vi "Mic Amps Sync.vi"() -> ()   [LabVIEW 2018, in "Impedance Tube.lvlib"]
uses:
  <vilib>/sound2/lvsound2.llb/Sound Data Format.ctl
  <vilib>/sound2/lvsound2.llb/Sampling Mode.ctl
  <vilib>/sound2/lvsound2.llb/Sound Output Set Volume (Single).vi
  <vilib>/sound2/lvsound2.llb/Sound Output Write (DBL Single).vi
  <vilib>/sound2/lvsound2.llb/Sound Input Read (DBL).vi
  <vilib>/addons/Sound and Vibration/svt_Level/SVT Sound Level (N Ch).vi
  Impedance Tube.lvlib
  <vilib>/measure/NI_MABase.lvlib
  <vilib>/addons/Sound and Vibration/svt_Level/SoundVib_SoundLevel.lvlib
panel:
  out "Scalar 2":dbl
  out "Scalar":dbl
  out "Filtered Signal 3":dynamicdata(graph) caption="Filtered Signal"
  out "Speaker Device":dbl
  out "Filtered Signal 2":dynamicdata(graph) caption="Filtered Signal"
  out "Mic B Device":dbl
  out "mv 2":dbl
  out "db B":dbl
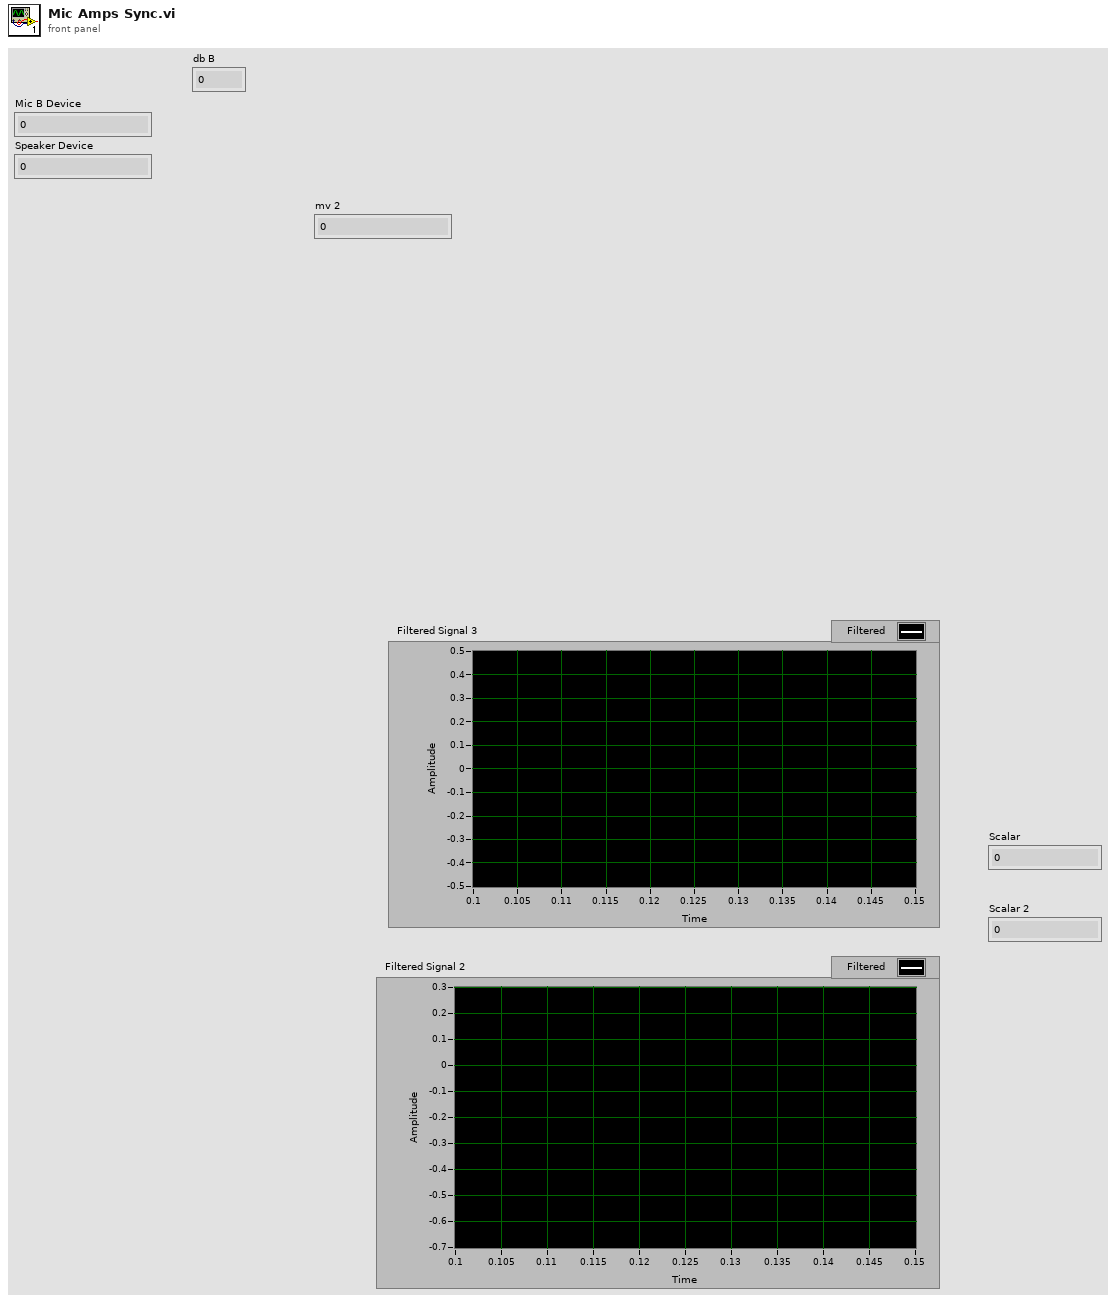
[diagram p1: front panel]
types:
  T1 = cluster{"Leq":bool, "Running Leq":bool, "Exponential":bool, "Peak":bool}
  T2 = typedef "Sound Data Format.ctl" = cluster{"sample rate (S/s)":dbl, "number of channels":i32, "bits per sample":i32}
  T3 = typedef "Sampling Mode.ctl" = i32
  T4 = typedef "Sound Output Task ID.ctl" = u32
  T5 = typedef "Sound Input Task ID.ctl" = u32
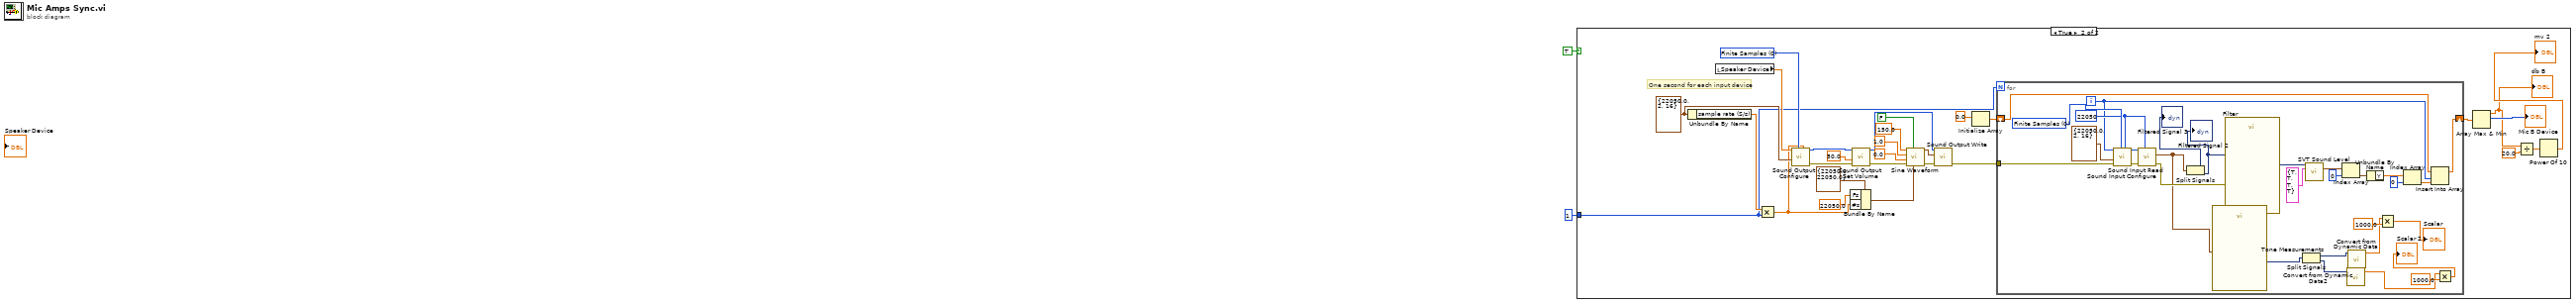
[diagram p0: block diagram]
diagram:
  n1 = case shown="True" TRUE {
    tunnel: 1 ("Number of Input Devices") -> [_ w8]
    frame False {
    }
    frame True {
      w31 = T3 0 items=["Finite Samples", "Continuous Samples"] ("sample mode")
      w18 = T2 {"sample rate (S/s)"=22050.0, "number of channels"=2, "bits per sample"=16} ("sound format")
      # "One second for each input device"
      n2 = Unbundle By Name(w18) -> ("sample rate (S/s)"=w17:dbl)
      n3 = local read "Speaker Device"() -> (w28:dbl)
      n4 = Multiply(x=w17, y=w8) -> (x*y=w15:dbl)
      n5 = call <vilib>:"Sound Output Configure.vi"("number of samples/ch"=w15, "sample mode"=w31, "sound format"=w18, "device ID"=w28) -> ("error out"=w29:errorcluster, "task ID"=w30:T4)  [unwired: 6 in]
      n6 = Bundle By Name(cluster=cluster{"Fs":dbl, "#s":dbl} {"Fs"=22050.0, "#s"=22050.0} ("sampling info"), "Fs"=22050.0, "#s"=w15) -> (w13:cluster{"Fs":dbl, "#s":dbl})
      n7 = call-poly <vilib>:"Sound Output Set Volume.vi"("error in (no error)"=w29, "volume"=50.0, "task ID"=w30) -> ("error out"=w23:errorcluster, "task ID out"=w27:T4)  [unwired: 7 in]
      n8 = call <vilib>:"Sine Waveform.vi"("sampling info"=w13, "reset signal"=FALSE, "error in (no error)"=w23, "phase"=0.0, "amplitude"=1.0, "frequency"=150.0) -> ("error out"=w22:errorcluster, "signal out"=w20:waveform(dbl))  [unwired: 4 in]
      n9 = call-poly <vilib>:"Sound Output Write.vi"("error in (no error)"=w22, "data"=w20, "task ID"=w27) -> ("error out"=w10:errorcluster)  [unwired: 7 in, 1 out]
      n10 = Initialize Array(0.0 ("element")) -> (w11:dbl[])  [unwired: 1 in]
      n11 = for {
        N: w8 -> [_]
        shift-right: [w49] -> w9
        shift-left: w11 -> [w50]
        tunnel: w10 -> [w46]
        i -> [w47]
        w57 = 22050 ("number of samples/ch")
        w60 = T3 0 items=["Finite Samples", "Continuous Samples"] ("sample mode")
        n12 = call <vilib>:"Sound Input Configure.vi"("number of samples/ch"=w57, "sample mode"=w60, "error in (no error)"=w46, "sound format"=T2 {"sample rate (S/s)"=22050.0, "number of channels"=2, "bits per sample"=16}, "device ID"=w47) -> ("error out"=w59:errorcluster, "task ID"=w58:T5)  [unwired: 5 in]
        n13 = call-poly <vilib>:"Sound Input Read.vi"("number of samples/ch"=w57, "error in (no error)"=w59, "task ID"=w58) -> ("error out"=w45:errorcluster, "data"=w41:waveform(dbl)[])  [unwired: 6 in, 1 out]
        n14 = Split Signals(w41) -> (→"Filtered Signal 3":dynamicdata, w43:dynamicdata)  [unwired: 2 in]
        "Filtered Signal 2" <- w43
        n15 = call "Tone Measurements"("Signals"=w41) -> ("Amplitude"=w40:dynamicdata)  [unwired: 9 in, 1 out]
        n16 = call "Filter"("error in (no error)"=w45, "Signal"=w43) -> ("Filtered Signal"=w44:dynamicdata)  [unwired: 8 in, 1 out]
        n17 = Split Signals(w40) -> (w39:dynamicdata, w38:dynamicdata)  [unwired: 2 in]
        n18 = call-poly <vilib>:"SVT Sound Level.vi"("scaled signals [EU]"=w44, "measurement selection"=T1 {"Leq"=TRUE, "Running Leq"=TRUE, "Exponential"=TRUE, "Peak"=TRUE}) -> ("running Leq sound levels [dB EU]"=w55:waveform(dbl)[])  [unwired: 8 in, 5 out]
        n19 = Index Array(array=w55, index=0) -> (element=w53:waveform(dbl))
        n20 = call "Convert from Dynamic Data2"("Dynamic Data Type"=w38) -> ("Scalar"=w35:dbl)  [unwired: 3 in]
        n21 = call "Convert from Dynamic Data"("Dynamic Data Type"=w39) -> ("Scalar"=w34:dbl)  [unwired: 3 in]
        n22 = Unbundle By Name(w53) -> ("Y"=w51:dbl[])
        n23 = Multiply(x=w34, y=1000.0) -> (x*y=→"Scalar":dbl)
        n24 = Index Array(array=w51, index=0) -> (element=w48:dbl)
        n25 = Insert Into Array(array=w50, index=w47, new element=w48) -> (w49:dbl[])
        n26 = Multiply(x=w35, y=1000.0) -> (x*y=→"Scalar 2":dbl)
      }
      n27 = Array Max & Min(array=w9) -> (max value=w3:dbl, max index (indices)=→"Mic B Device":i32)  [unwired: 2 out]
      "db B" <- w3
      n28 = Divide(x=w3, y=20.0) -> (x/y=w6:dbl)
      n29 = Power Of 10(x=w6) -> (10^x=→"mv 2":dbl)
    }
  }
